vi "Write position in AI tasks.vi"(8 "error in (no error)":errorcluster, 10 "position in AI tasks":dbl, 11 "DAQmxTaskAIVoltage_General in":refnum<class "DAQmxTaskAIVoltage_General.lvclass">) -> (0 "error out":errorcluster, 3 "DAQmxTaskAIVoltage_General out":refnum<class "DAQmxTaskAIVoltage_General.lvclass">)   [LabVIEW 2019, in "DAQmxTaskAIVoltage_General.lvclass"]
uses:
  DAQmxTaskAIVoltage_General.lvclass
  DAQmxTaskAIVoltage_General.lvclass/DAQmxTaskAIVoltage_General.ctl
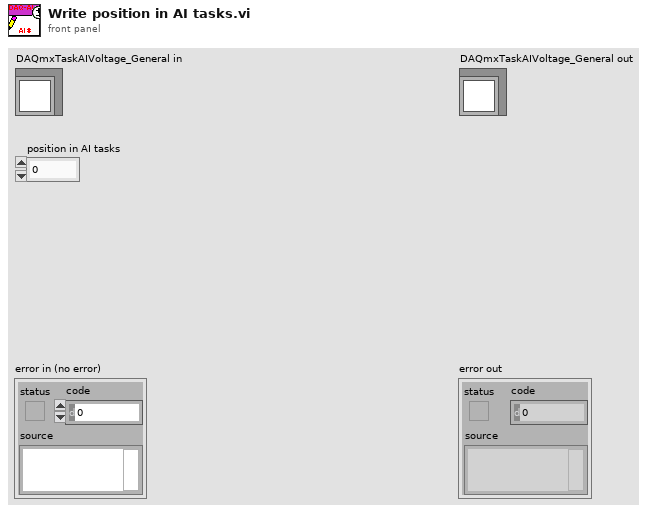
[diagram p1: front panel]
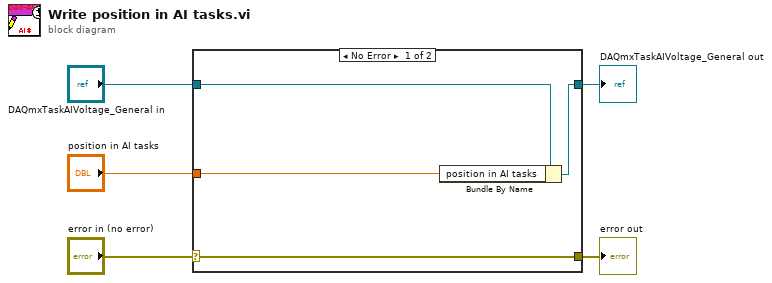
[diagram p0: block diagram]
diagram:
  n1 = case shown="No Error" "error in (no error)" {
    selector: "error in (no error)" -> [w9 w10]
    tunnel: [w9 w10] -> w4
    tunnel: [w7 w11] -> w2
    tunnel: "DAQmxTaskAIVoltage_General in" -> [w8 w11]
    tunnel: "position in AI tasks" -> [w6 _]
    frame No Error {
      n2 = Bundle By Name(cluster=w8, "position in AI tasks"=w6) -> (w7:refnum<class "DAQmxTaskAIVoltage_General.lvclass">)
    }
    frame Error {
    }
  }
  "error out" <- w4
  "DAQmxTaskAIVoltage_General out" <- w2
